vi "FocusOptimization.vi"   [LabVIEW 2019]
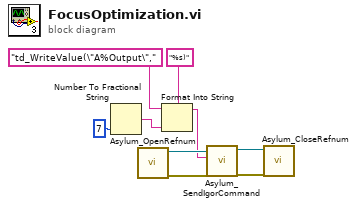
[diagram p0: block diagram]
diagram:
  n1 = Number To Fractional String(precision (6)=i16 7) -> (number=w6:dbl, F-format string=w3:string)  [unwired: 2 in]
  n2 = call <vilib>:"Asylum_OpenRefnum.vi"() -> ("error out"=w10:errorcluster, "Application"=w8:refnum<k7>)  [unwired: 10 in]
  n3 = Format Into String(format string="%s)" ("string"), initial string="td_WriteValue(\"A%Output\"," ("string"), w3) -> (resulting string=w1:string)  [unwired: 1 in, 1 out]
  n4 = call <vilib>:"Asylum_SendIgorCommand.vi"("error in (no error)"=w10, "command"=w1, "Application"=w8) -> ("error out"=w9:errorcluster, "Application"=w7:refnum<k7>)  [unwired: 5 in, 2 out]
  n5 = call <vilib>:"Asylum_CloseRefnum.vi"("error in (no error)"=w9, "Application"=w7) -> ()  [unwired: 9 in, 1 out]
